vi "IN-20-en_velosim.vi"() -> ()   [LabVIEW 2010]
uses:
  Instance           1 20Saved   exo_velo_cor .vi
panel:
  out "Temps total en mn":dbl format="%.2f"
  out "Distance cumulée en Km":dbl format="%.2f"
  in  "stop":bool
  out "Vitesse moyenne\nen Km/h":dbl format="%.2f"
  out "Vitesse instantanée":dbl(knob) scale=0.0..80.0
  in  "Fréquence de pédalage en tr/mn":dbl(knob)=20.0 min=20.0 max=180.0 step=5.0 scale=0.0..150.0 scale format="%.1f"
  in  "Plateau avant":i8(knob)=30 min=30 max=55 step=1 scale=30.0..55.0
  in  "Pignon arrière":i8(knob)=13 min=11 max=32 step=1 scale=11.0..26.0
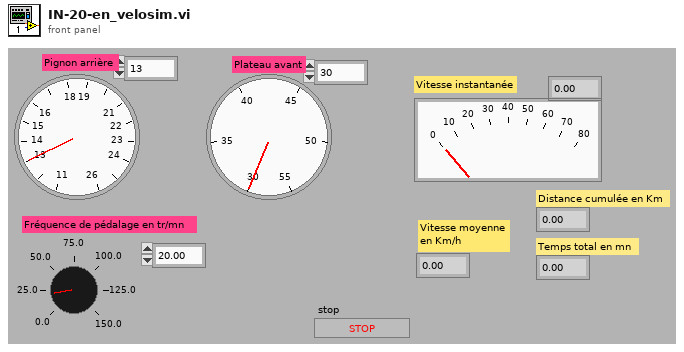
[diagram p1: front panel]
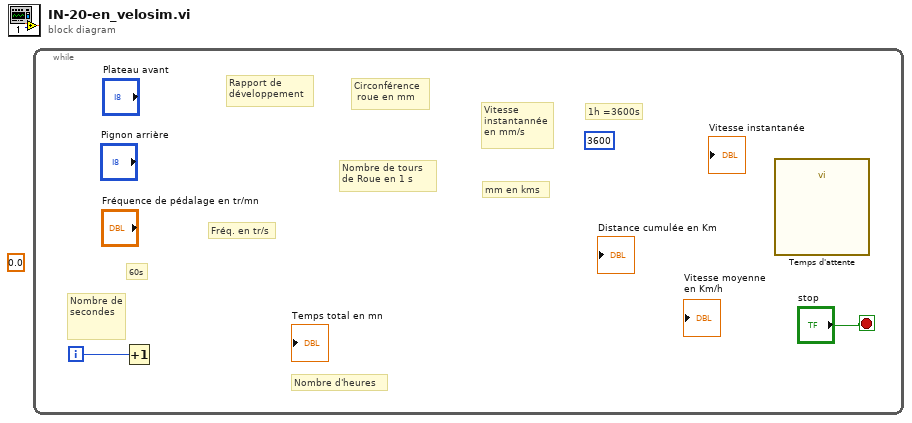
[diagram p0: block diagram]
diagram:
  (unwired) 0.0
  n1 = while {
    i -> [w1]
    stop <- "stop" stop-if-true
    (unwired) 3600
    # "mm en kms"
    # "1h =3600s"
    # "Nombre d'heures"
    # "Nombre de secondes"
    # "Vitesse instantannée\nen mm/s"
    # "Nombre de tours \nde Roue en 1 s"
    # "Rapport de \ndéveloppement"
    # "60s"
    # "Fréq. en tr/s"
    # "Circonférence\n roue en mm"
    n2 = Increment(x=w1) -> ()  [unwired: 1 out]
    n3 = call "Temps d'attente"() -> ()  [unwired: 11 in, 1 out]
  }
